vi "Host - DRAM FIFO test.vi"() -> ()   [LabVIEW 2019]
uses:
  <vilib>/userdefined/High Color/nirio_resource_hc.ctl
  <vilib>/FPGAPlugInAG/PXIe-7902R/niLvFpga_Open_PXIe-7902R.vi
  <vilib>/rvi/interface/common/dynamic/niFpgaDynamicAddResources.vi
  <vilib>/Utility/error.llb/Error Cluster From Error Code.vi
  <vilib>/rvi/errors/niLvFpgaAdjustHostInterfaceError.vi
  <vilib>/rvi/interface/common/niFpgaWaitOnOcc.vi
  <vilib>/FPGAPlugInAG/Dynamic/niLvFpga_Close_Dynamic.vi
  <vilib>/rvi/interface/nirviOpenFPGA/nirviOpenFPGA.xnode
  FPGA Bitfiles/barkhausenmmwave_ReceiveFPGA(3.07_DRAMFIFOtest_t4Z5IoaW5Fs.lvbitx
  <vilib>/rvi/interface/nirviReadWriteControl/nirviReadWriteControl.xnode
  <vilib>/rvi/interface/nirviMethod/nirviMethod.xnode
  <vilib>/rvi/interface/nirviCloseFPGA/nirviCloseFPGA.xnode
  NiFpgaLv.dll
  <vilib>/rvi/interface/Simulation/niFpgaSimulationCallBeginRW.vi
  <vilib>/FPGAPlugInAG/Dynamic/niLvFpga_ConfigureFifo_Dynamic.vi
  <vilib>/rvi/errors/niLvFpgaMergeErrorWithErrorCode.vi
  <vilib>/FPGAPlugInAG/Dynamic/niLvFpga_ReadFifo_Dynamic.vi
  <vilib>/FPGAPlugInAG/Dynamic/niLvFpga_WriteFifo_Dynamic.vi
panel:
  out "size(s)":i32
  out "fixed-point":fxp<+/-,16,1>
  out "DRAM highwater":u32
  out "Output data 2":fxp<+/-,16,1>[](array[numeric])
  in  "I":fxp<+/-,16,1>
  out "status":T1
  out "Output data":fxp<+/-,16,1>[](array[numeric])
  in  "Stop Button":bool
  in  "read":bool
  out "Elements Remaining":u32
  in  "repeat":i32
  in  "Input data":fxp<+/-,16,1>[](array[numeric])
  in  "resource name":T2
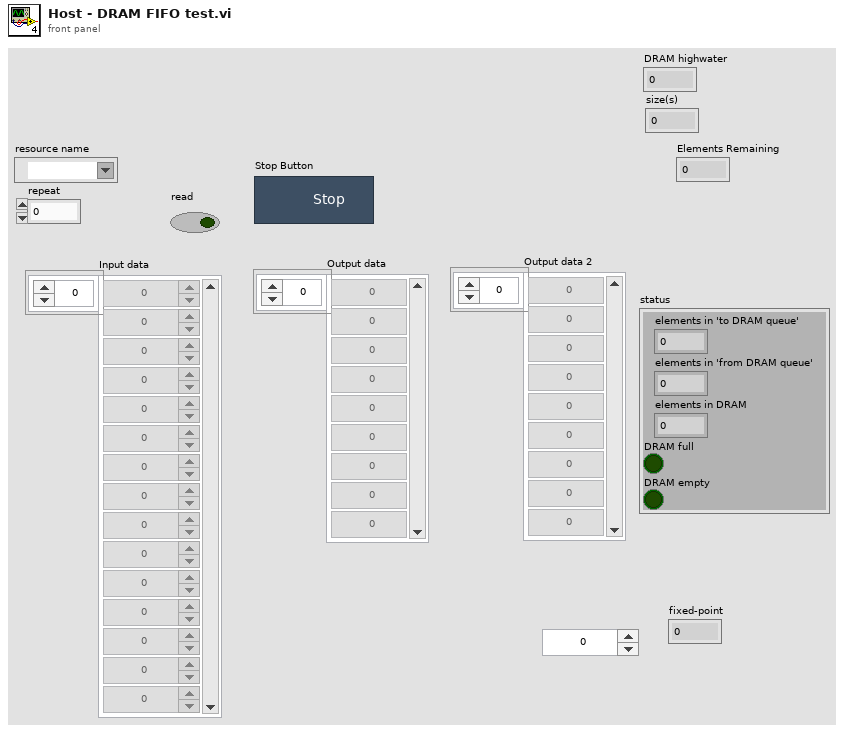
[diagram p1: front panel]
types:
  T1 = cluster{"elements in 'to DRAM queue'":u32, "elements in 'from DRAM queue'":u32, "elements in DRAM":u32, "DRAM full":bool, "DRAM empty":bool}
  T2 = typedef "nirio_resource_hc.ctl" = tag
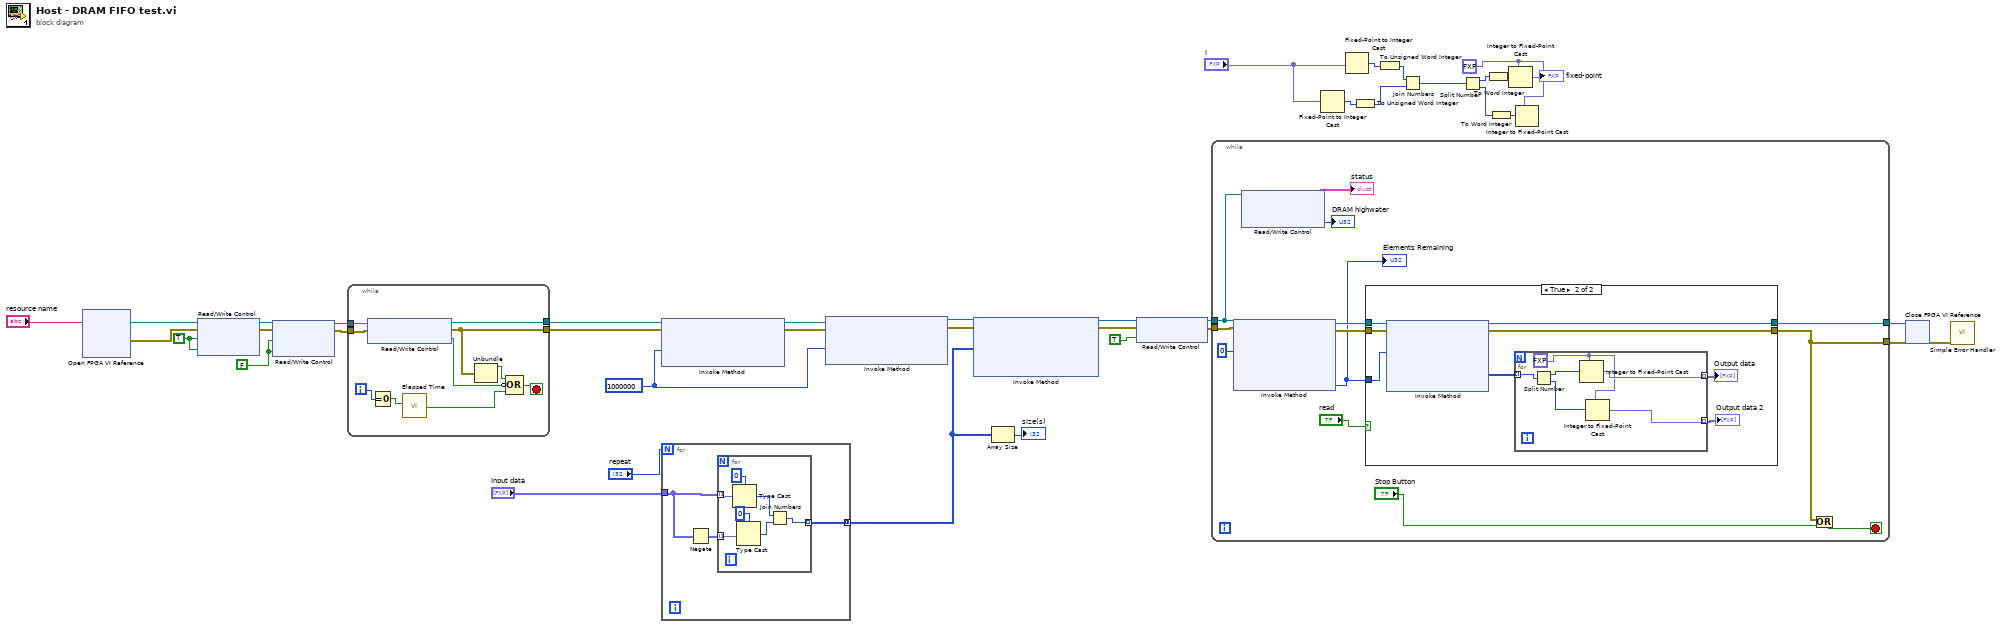
[diagram p0: block diagram]
diagram:
  w7 = fxp<+/-,16,1> 0.0 ("number")
  w28 = u32 1000000 ("Requested Depth")
  w34 = FALSE ("reset")
  w38 = TRUE ("reset")
  n1 = xnode "Open FPGA VI Reference"("resource name"="resource name") -> ("FPGA VI Reference Out"=w39:refnum<k20>, "error out"=w37:errorcluster)  [unwired: 1 in]
  n2 = xnode "Read/Write Control"("FPGA VI Reference In"=w39, "error in"=w37, "reset"=w38, "reset DRAM"=w38) -> ("FPGA VI Reference Out"=w36:refnum<k20>, "error out"=w35:errorcluster)
  n3 = xnode "Read/Write Control"("FPGA VI Reference In"=w36, "error in"=w35, "reset"=w34, "reset DRAM"=w34) -> ("FPGA VI Reference Out"=w33:refnum<k20>, "error out"=w32:errorcluster)
  n4 = while {
    tunnel: w33 -> [w50]
    tunnel: w32 -> [w43]
    tunnel: [w42] -> w31
    tunnel: [w41] -> w30
    i -> [w46]
    stop <- w48 stop-if-true
    n5 = xnode "Read/Write Control"("FPGA VI Reference In"=w50, "error in"=w43) -> ("FPGA VI Reference Out"=w42:refnum<k20>, "error out"=w41:errorcluster, "reset in progress?"=w49:bool)
    n6 = Equal To 0?(x=w46) -> (x = 0?=w45:bool)
    n7 = call "Elapsed Time"("Reset"=w45) -> ("Time has Elapsed"=w44:bool)  [unwired: 11 in, 7 out]
    n8 = Unbundle(w41) -> ("status"=w47:bool)  [unwired: 2 out]
    n9 = Compound Arithmetic op=OR(w47, invert w49, w44) -> (w48:bool)
  }
  n10 = xnode "Invoke Method"("FPGA VI Reference In"=w31, "error in"=w30, "Requested Depth"=w28) -> ("FPGA VI Reference Out"=w29:refnum<k20>, "error out"=w27:errorcluster)  [unwired: 1 out]
  n11 = for {
    N: "repeat" -> [_]
    tunnel: "Input data" -> [w53]
    tunnel: [w51] -> w2 mode=concatenating
    n12 = Negate(x=w53) -> (-x=w52:fxp<+/-,17,2>[])
    n13 = for {
      tunnel: w53 -> [w60] mode=indexing
      tunnel: w52 -> [w57] mode=indexing
      tunnel: [w54] -> w51 mode=indexing
      n14 = Type Cast(type=u16 0, x=w60) -> (*(type *) &x=w55:u16)
      n15 = Type Cast(type=u16 0, x=w57) -> (*(type *) &x=w56:u16)
      n16 = Join Numbers(hi=w55, lo=w56) -> ((hi.lo)=w54:u32)
    }
  }
  n17 = xnode "Invoke Method"("FPGA VI Reference In"=w29, "error in"=w27, "Requested Depth"=w28) -> ("FPGA VI Reference Out"=w26:refnum<k20>, "error out"=w25:errorcluster)  [unwired: 1 out]
  n18 = xnode "Invoke Method"("FPGA VI Reference In"=w26, "error in"=w25, "Data"=w2) -> ("FPGA VI Reference Out"=w23:refnum<k20>, "error out"=w18:errorcluster)  [unwired: 1 in, 1 out]
  n19 = Array Size(array=w2) -> (size(s)=→"size(s)":i32)
  n20 = xnode "Read/Write Control"("FPGA VI Reference In"=w23, "error in"=w18, "enable stream"=TRUE) -> ("FPGA VI Reference Out"=w19:refnum<k20>, "error out"=w17:errorcluster)
  n21 = while {
    tunnel: w19 -> [w64]
    tunnel: [w66] -> w22
    tunnel: [w65] -> w21
    tunnel: w17 -> [w62]
    stop <- w71 stop-if-true
    n22 = xnode "Invoke Method"("FPGA VI Reference In"=w64, "error in"=w62, "Number of Elements"=u32 0) -> ("FPGA VI Reference Out"=w69:refnum<k20>, "error out"=w68:errorcluster, "Elements Remaining"=w67:u32)  [unwired: 1 in, 1 out]
    "Elements Remaining" <- w67
    n23 = xnode "Read/Write Control"("FPGA VI Reference In"=w64) -> ("status"=→"status":T1, "DRAM highwater"=→"DRAM highwater":u32)  [unwired: 1 in, 2 out]
    n24 = case shown="True" "read" {
      tunnel: w69 -> [w74 w83]
      tunnel: w68 -> [w75 w82]
      tunnel: [w75 w81] -> w65
      tunnel: w67 -> [_ w79]
      tunnel: [w74 w78] -> w66
      frame False {
      }
      frame True {
        n25 = xnode "Invoke Method"("FPGA VI Reference In"=w83, "error in"=w82, "Number of Elements"=w79) -> ("FPGA VI Reference Out"=w78:refnum<k20>, "error out"=w81:errorcluster, "Data"=w80:u32[])  [unwired: 1 in, 1 out]
        n26 = for {
          tunnel: w80 -> [w89] mode=indexing
          tunnel: [w86] -> w77 mode=indexing
          tunnel: [w88] -> w76 mode=indexing
          w85 = fxp<+/-,12,1> 0.0 ("number")
          n27 = Split Number(x=w89) -> (hi(x)=w84:u16, lo(x)=w87:u16)
          n28 = Integer to Fixed-Point Cast(fixed-point type=w85, integer=w84) -> (fixed-point=w88:fxp<+/-,12,1>)
          n29 = Integer to Fixed-Point Cast(fixed-point type=w85, integer=w87) -> (fixed-point=w86:fxp<+/-,12,1>)
        }
        "Output data" <- w76
        "Output data 2" <- w77
      }
    }
    n30 = Or(x=w65, y="Stop Button") -> (x .or. y?=w71:bool)
  }
  n31 = Fixed-Point to Integer Cast(1:"I") -> (0:w13:i16)
  n32 = Fixed-Point to Integer Cast(1:"I") -> (0:w14:i16)
  n33 = To Unsigned Word Integer(number=w13) -> (unsigned 16bit integer=w12:u16)
  n34 = To Unsigned Word Integer(number=w14) -> (unsigned 16bit integer=w11:u16)
  n35 = Join Numbers(hi=w11, lo=w12) -> ((hi.lo)=w4:u32)
  n36 = Split Number(x=w4) -> (hi(x)=w5:u16, lo(x)=w6:u16)
  n37 = To Word Integer(number=w5) -> (16bit integer=w8:i16)
  n38 = To Word Integer(number=w6) -> (16bit integer=w9:i16)
  n39 = Integer to Fixed-Point Cast(fixed-point type=w7, integer=w8) -> (fixed-point=→"fixed-point":fxp<+/-,16,1>)
  n40 = Integer to Fixed-Point Cast(fixed-point type=w7, integer=w9) -> ()  [unwired: 1 out]
  n41 = xnode "Close FPGA VI Reference"("FPGA VI Reference In"=w22, "error in"=w21) -> ("error out"=w20:errorcluster)
  n42 = call <vilib>:"Simple Error Handler.vi"("error in (no error)"=w20) -> ()  [unwired: 4 in, 5 out]
